vi "Read elements.vi"(8 "error in (no error)":errorcluster, 11 "Topic in":refnum<class "Topic.lvclass">) -> (0 "error out":errorcluster, 2 "elements":refnum<class "Element.lvclass">[](array[class]), 3 "Topic out":refnum<class "Topic.lvclass">)   [LabVIEW 2018, in "Topic.lvclass"]
doc: "Read the elements."
uses:
  Topic.lvclass
  Element/Element.lvclass
  Topic.lvclass/Topic.ctl
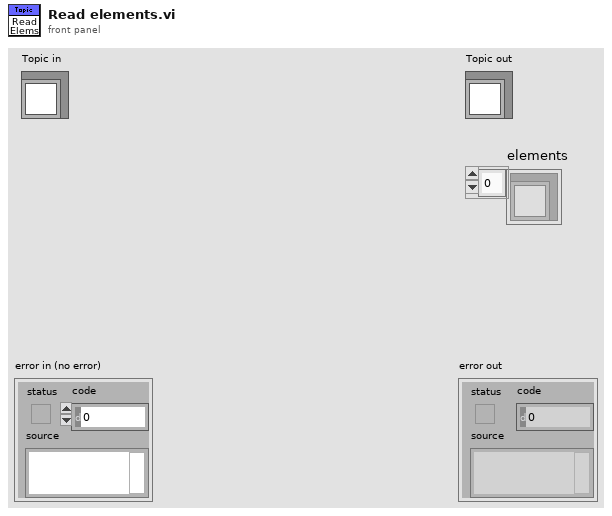
[diagram p1: front panel]
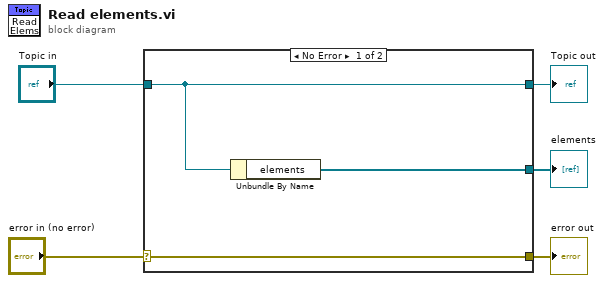
[diagram p0: block diagram]
diagram:
  n1 = case shown="No Error" "error in (no error)" {
    selector: "error in (no error)" -> [w8 w9]
    tunnel: [w8 w9] -> w4
    tunnel: [w7 w10] -> w2
    tunnel: "Topic in" -> [w7 w10]
    tunnel: [w6 _] -> w1
    frame No Error {
      n2 = Unbundle By Name(w7) -> ("elements"=w6:refnum<class "Element.lvclass">[])
    }
    frame Error {
    }
  }
  "error out" <- w4
  "Topic out" <- w2
  "elements" <- w1
